vi "Add_or_replace_chan.vi"(4 "Fiirst call":bool, 6 "Interactive":bool=TRUE, 7 "group name":string="Untitled", 8 "Error In":errorcluster, 9 "Add to channel list":string, 10 "Waveforms":waveform(dbl)[](array[waveform]), 11 "File Path Control":path) -> (0 "Error Out":errorcluster, 1 "channel name(s) out":string[](array[string]), 2 "group name out":string, 3 "file path out":path)   [LabVIEW 2015]
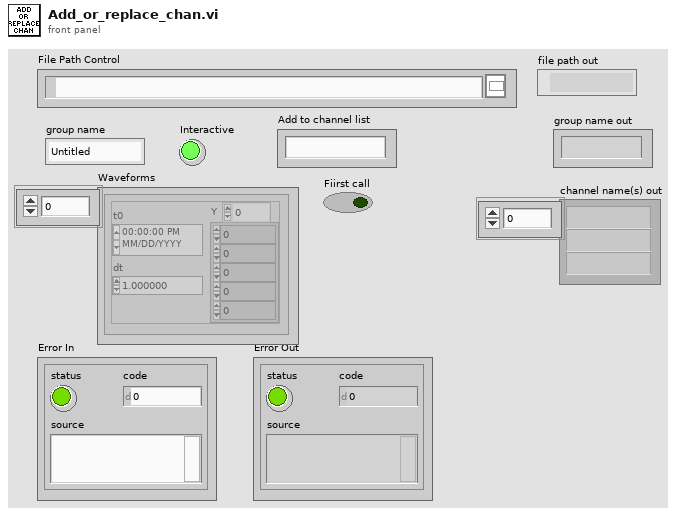
[diagram p1: front panel]
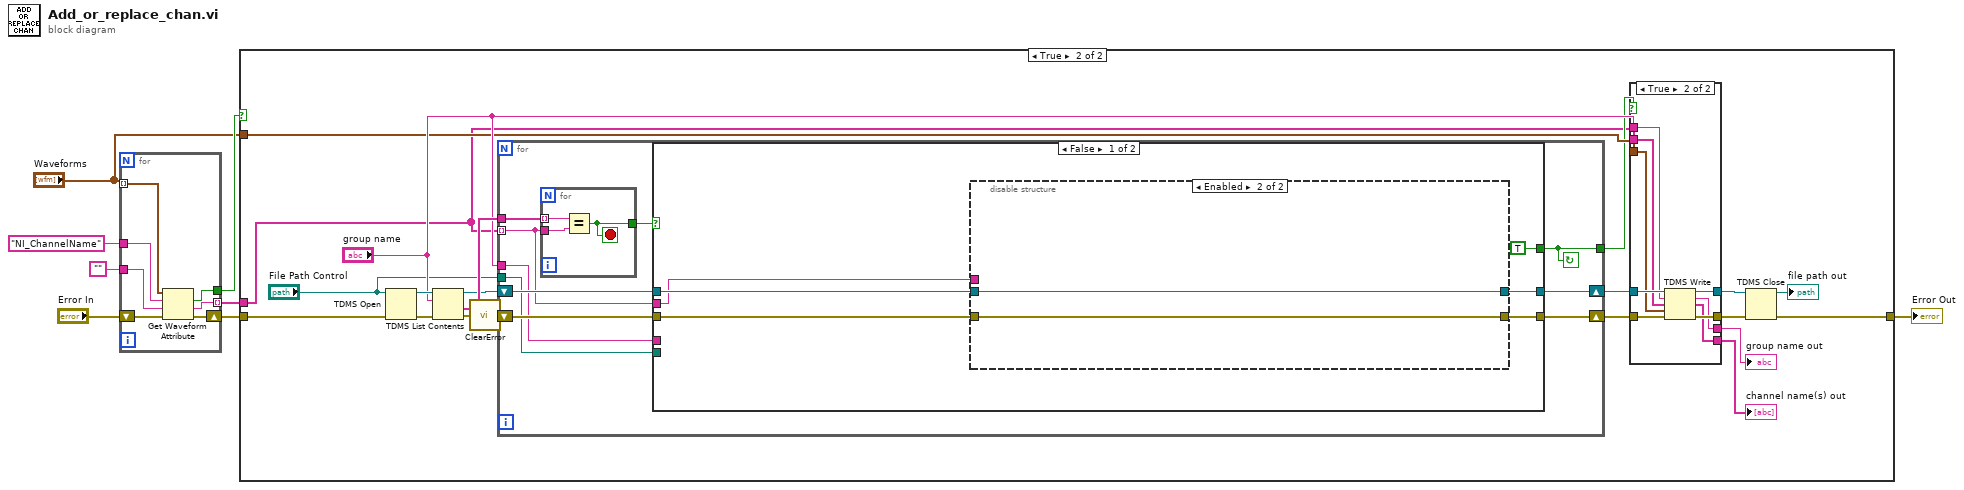
[diagram p0: block diagram]
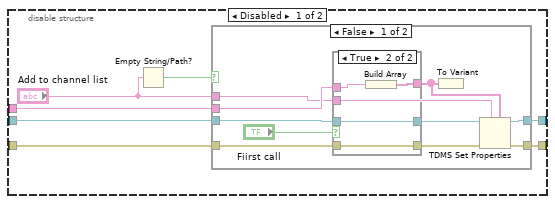
[diagram p3: hidden frame]
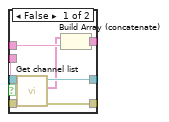
[diagram p4: hidden frame]
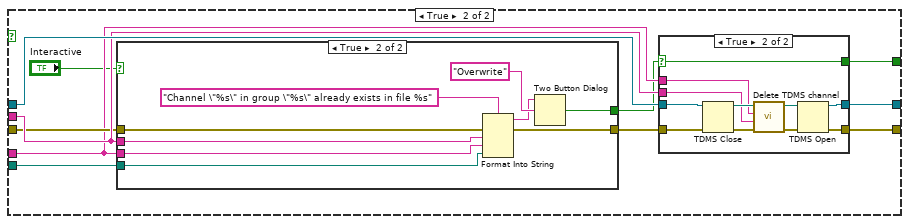
[diagram p6: hidden frame]
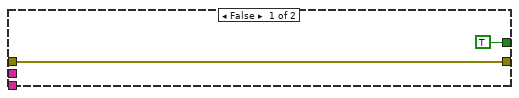
[diagram p7: hidden frame]
diagram:
  n1 = for {
    tunnel: [w14] -> w7
    tunnel: [w12] -> w5 mode=indexing
    tunnel: "Waveforms" -> [w11] mode=indexing
    shift-right: [w13] -> w6
    shift-left: "Error In" -> [w15]
    tunnel: "NI_ChannelName" ("name") -> [w10]
    tunnel: "" -> [w9]
    n2 = Get Waveform Attribute(4:w15, 5:w9, 6:w10, 7:w11) -> (0:w13:errorcluster, 1:w12:string, 2:w14:bool)  [unwired: 1 out]
  }
  n3 = case shown="True" w7 {
    tunnel: w6 -> [w16 w36]
    tunnel: w5 -> [_ w20]
    tunnel: "Waveforms" -> [_ w28]
    tunnel: [w16 w24] -> w4
    frame False {
    }
    frame True {
      n4 = TDMS Open(8:w36, 11:"File Path Control") -> (0:w35:errorcluster, 3:w34:refnum<k34>)  [unwired: 5 in]
      n5 = TDMS List Contents(4:w35, 6:"group name", 7:w34) -> (0:w17:errorcluster, 1:w33:string[], 3:w32:refnum<k34>)  [unwired: 1 out]
      n6 = call <vilib>:"ClearError.vi"("error in (no error)"=w17) -> ("error out"=w31:errorcluster)
      n7 = for {
        tunnel: w33 -> [w46]
        tunnel: "group name" -> [w41]
        tunnel: w20 -> [w40] mode=indexing
        tunnel: [w37] -> w23
        tunnel: "File Path Control" -> [w38]
        shift-right: [w42] -> w30
        shift-left: w32 -> [w45]
        shift-right: [w39] -> w27
        shift-left: w31 -> [w44]
        stop <- w37 continue-if-true
        n8 = for {
          tunnel: w46 -> [w124] mode=indexing
          tunnel: w40 -> [w123]
          tunnel: [w122] -> w43
          stop <- w122 stop-if-true
          n9 = Equal?(x=w124, y=w123) -> (x = y?=w122:bool)
        }
        n10 = case shown="False" w43 {
          tunnel: w45 -> [w51 w96]
          tunnel: w44 -> [w50 w91]
          tunnel: [w48 w95] -> w39
          tunnel: [w49 w94] -> w42
          tunnel: w41 -> [_ w89]
          tunnel: w40 -> [w47 w92]
          tunnel: [TRUE w93] -> w37
          tunnel: w38 -> [_ w88]
          frame False {
            n11 = disable-structure shown="Enabled" {
              disable-tunnel: w51 -> [w59 w84]
              disable-tunnel: w50 -> [w58 w85]
              disable-tunnel: [w57 w84] -> w49
              disable-tunnel: [w56 w85] -> w48
              disable-tunnel: w47 -> [w55 _]
              frame Disabled {
                n12 = Empty String/Path?(string/path="Add to channel list") -> (empty?=w53:bool)
                n13 = case shown="False" w53 {
                  tunnel: w59 -> [w67 w83]
                  tunnel: w58 -> [w64 w82]
                  tunnel: [w69 w83] -> w57
                  tunnel: [w68 w82] -> w56
                  tunnel: w55 -> [w63 _]
                  tunnel: "Add to channel list" -> [w62 _]
                  frame False {
                    n14 = case shown="True" "Fiirst call" {
                      tunnel: [w77 w81] -> w60
                      tunnel: w67 -> [w76 w79]
                      tunnel: [w75 w79] -> w66
                      tunnel: [w74 w78] -> w65
                      tunnel: w64 -> [w73 w78]
                      tunnel: w63 -> [w72 w80]
                      tunnel: w62 -> [w70 _]
                      frame False {
                        n15 = call "Get channel list.vi"("Error In"=w73, "Channel list"=w70, "tdms file"=w76) -> ("Error Out"=w74:errorcluster, "Array - String"=w71:string[], "tdms file out"=w75:refnum<k34>)  [unwired: 6 in]
                        n16 = Build Array (concatenate)(w71, w72) -> (w77:string[])
                      }
                      frame True {
                        n17 = Build Array(w80) -> (w81:string[])
                      }
                    }
                    n18 = To Variant(anything=w60) -> ()  [unwired: 1 out]
                    n19 = TDMS Set Properties(5:w60, 7:w62, 8:w65, 11:w66) -> (0:w68:errorcluster, 3:w69:refnum<k34>)  [unwired: 2 in, 2 out]
                  }
                  frame True {
                  }
                }
              }
              frame Enabled {
              }
            }
          }
          frame True {
            n20 = case shown="True" "Interactive" {
              tunnel: w92 -> [_ w103]
              tunnel: w91 -> [w98 w105]
              tunnel: [w98 w104] -> w90
              tunnel: w89 -> [_ w102]
              tunnel: w88 -> [_ w101]
              tunnel: [TRUE ("T button?") w100] -> w86
              frame False {
              }
              frame True {
                n21 = Format Into String(format string="Channel \"%s\" in group \"%s\" already exists in file %s" ("string"), error in=w105, w103, w102, w101) -> (resulting string=w99:string, error out=w104:errorcluster)  [unwired: 1 in]
                n22 = Two Button Dialog(message=w99, 2:"Overwrite" ("T button name (\"OK\")")) -> (T button?=w100:bool)  [unwired: 1 in]
              }
            }
            n23 = case shown="True" w86 {
              selector: w86 -> [w109 w111]
              tunnel: w96 -> [w108 w121]
              tunnel: w90 -> [w110 w118]
              tunnel: [w110 w115] -> w95
              tunnel: [w108 w114] -> w94
              tunnel: w89 -> [_ w113]
              tunnel: w92 -> [_ w112]
              tunnel: [w109 w111] -> w93
              frame False {
              }
              frame True {
                n24 = TDMS Close(8:w118, 11:w121) -> (0:w119:errorcluster, 3:w120:path)
                n25 = call "Delete TDMS channel.vi"("Error In"=w119, "Channel"=w112, "Group"=w113, "Source Path"=w120) -> ("Error Out"=w117:errorcluster, "Source Path out"=w116:path)  [unwired: 6 in]
                n26 = TDMS Open(8:w117, 11:w116) -> (0:w115:errorcluster, 3:w114:refnum<k34>)  [unwired: 5 in]
              }
            }
          }
        }
      }
      n27 = case shown="True" w23 {
        tunnel: w30 -> [w128 w137]
        tunnel: "group name" -> [w126 w136]
        tunnel: w28 -> [_ w135]
        tunnel: w27 -> [w127 w134]
        tunnel: [w127 w133] -> w26
        tunnel: [w128 w132] -> w25
        tunnel: w20 -> [w125 w131]
        tunnel: [w126 w130] -> w19
        tunnel: [w125 w129] -> w18
        frame False {
        }
        frame True {
          n28 = TDMS Write(0:w137, 5:w136, 7:w131, 9:w135, 11:w134) -> (4:w132:refnum<k34>, 6:w130:string, 8:w129:string[], 15:w133:errorcluster)  [unwired: 1 in]
        }
      }
      "group name out" <- w19
      "channel name(s) out" <- w18
      n29 = TDMS Close(8:w26, 11:w25) -> (0:w24:errorcluster, 3:→"file path out":path)
    }
  }
  "Error Out" <- w4
